vi "test_turbo2.vi"() -> ()   [LabVIEW 2018]
uses:
  <vilib>/addons/Modulation/Analog/support/mod_Set Error Source.vi
  <vilib>/addons/Modulation/Digital/Support/Common/Validators/mod_AWGN Validate.vi
  <vilib>/addons/Modulation/Digital/Impairments/subVIs/mod_createSeeds.vi
  <vilib>/addons/Modulation/Digital/Support/Common/Validators/mod_Validate Samples Per Symbol.vi
  <vilib>/addons/Modulation/Analog/support/Validators/mod_Validate Complex Waveform.vi
  <vilib>/addons/Modulation/Analog/support/Validators/mod_WFErrorHandler.vi
  <vilib>/addons/Modulation/Digital/Support/Common/Validators/mod_Generate Filter Coefficients Validate.vi
  <vilib>/addons/Modulation/Digital/General/subVIs/mod_Generate Filter Coefficients.vi
  <vilib>/addons/Modulation/Digital/General/MT Generate PSK System Parameters(M).vi
  <vilib>/addons/Modulation/Digital/General/subVIs/mod_Generate Bits PN Sequence.vi
  <vilib>/Analysis/1siggen.llb/Gaussian White Noise (obs 90).vi
  <vilib>/addons/Modulation/Digital/General/MT Apply Matched Filter (Generic).vi
  <vilib>/addons/Modulation/niDMT.lvlib
panel:
  out "message":i8[](array[numeric])
  out "#err":i32
  out "trial":i32
  in  "#trials":i32
  out "#bits":i32
  in  "Eb/N0":dbl=10.0 format="%.2f"
  out "BER":dbl
  out "Dec":i8[](array[numeric])
  out "sigma2":string
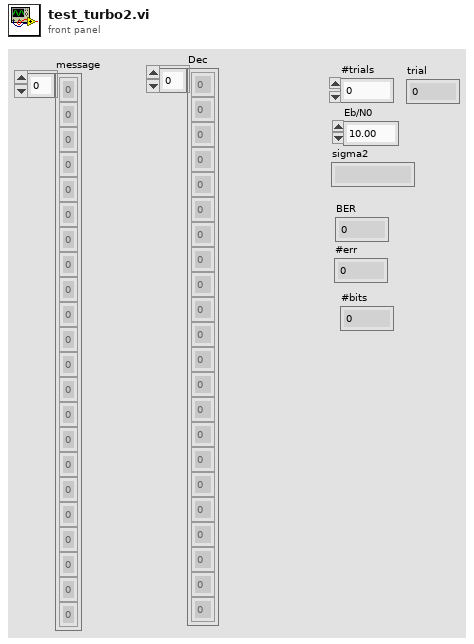
[diagram p1: front panel]
types:
  T1 = enum16{"none", "Raised Cosine", "Root Raised Cos", "Gaussian"}
  T2 = cluster{"samples per symbol (16)":i32, "symbol map":cdb[], "differential PSK":enum16{"disable", "enable"}, "PSK type":u16}
  T3 = typedef "niAMT.lvlib/Complex Data Waveform.ctl" = cluster{"t0":dbl, "dt":dbl, "Y":cdb[]}
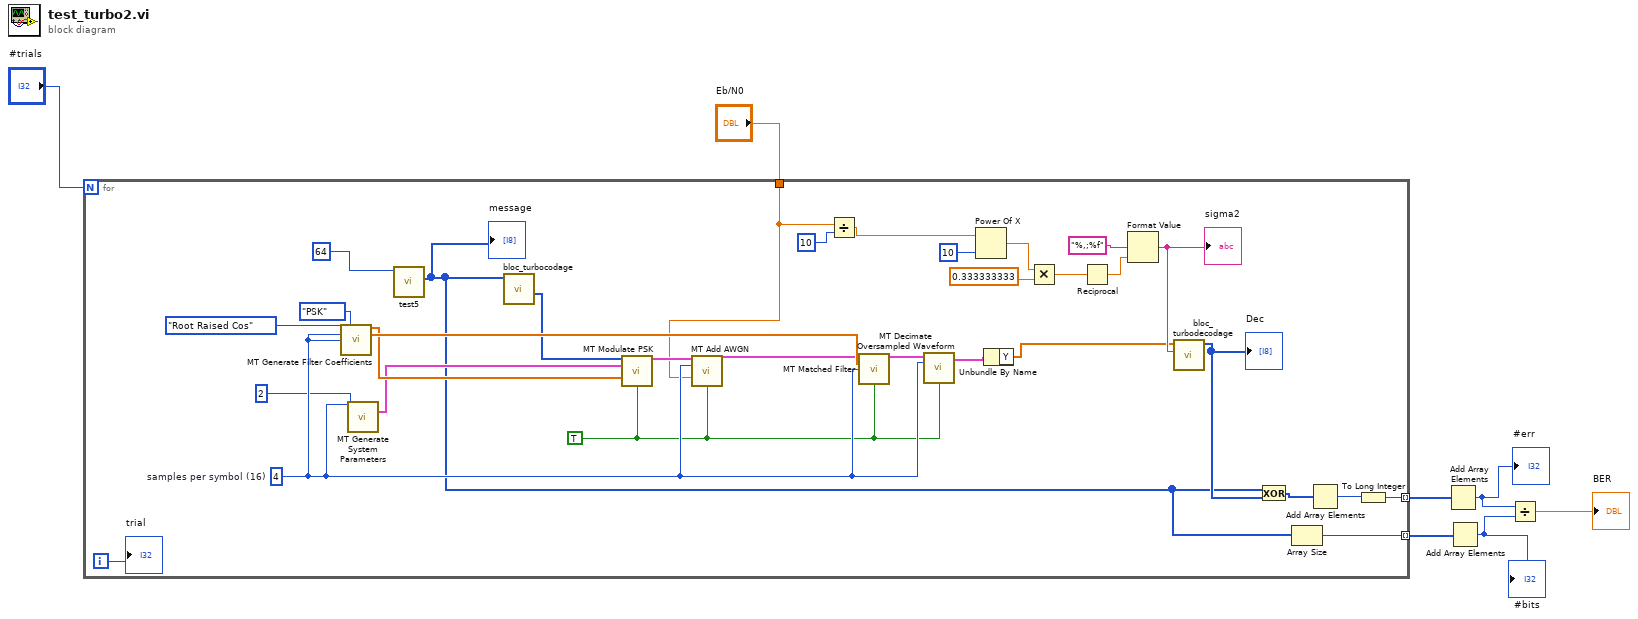
[diagram p0: block diagram]
diagram:
  n1 = for {
    N: "#trials" -> [_]
    tunnel: [w34] -> w6 mode=indexing
    tunnel: "Eb/N0" -> [w10]
    tunnel: [w25] -> w2 mode=indexing
    i -> [w27]
    w18 = 4  # samples per symbol (16)
    w14 = TRUE ("reset? (T)")
    n2 = call <vilib>:"MT Generate Filter Coefficients.vi"("pulse shaping filter (none)"=T1."Root Raised Cos", "modulation type"=enum16{"FSK", "PSK", "QAM", "MSK", "PAM", "ASK"}."PSK", "pulse shaping samples per symbol (16)"=w18, "matched samples per symbol (16)"=w18) -> ("pulse shaping filter coefficients"=w22:dbl[], "matched filter coefficients"=w24:dbl[])  [unwired: 9 in, 1 out]
    n3 = call-poly <vilib>:"MT Generate System Parameters.vi"("samples per symbol (16)"=w18, "M-PSK (4)"=2) -> ("PSK system parameters"=w19:T2)  [unwired: 11 in, 2 out]
    n4 = call "test5.vi"("k"=64) -> ("output bit stream"=w8:i8[])  [unwired: 9 in, 1 out]
    "message" <- w8
    n5 = call "bloc_turbocodage.vi"("Array in"=w8) -> ("output bit stream"=w21:i8[])  [unwired: 8 in, 2 out]
    n6 = call <vilib>:"MT Modulate PSK.vi"("input bit stream"=w21, "PSK system parameters"=w19, "pulse shaping filter coefficients"=w22, "reset? (T)"=w14) -> ("output complex waveform"=w23:T3)  [unwired: 9 in, 2 out]
    n7 = call <vilib>:"MT Add AWGN.vi"("input complex waveform"=w23, "samples per symbol (16)"=w18, "Eb/N0 (10 dB)"=w10, "reset? (T)"=w14) -> ("output complex waveform"=w11:T3)  [unwired: 9 in, 2 out]
    n8 = Divide(x=w10, y=10) -> (x/y=w29:dbl)
    n9 = call-poly <vilib>:"MT Matched Filter.vi"("input complex waveform"=w11, "matched filter coefficients"=w24, "samples per symbol (16)"=w18, "reset? (T)"=w14) -> ("output complex waveform"=w20:T3)  [unwired: 10 in, 1 out]
    n10 = call <vilib>:"MT Decimate Oversampled Waveform.vi"("input complex waveform"=w20, "decimation factor"=w18, "reset? (T)"=w14) -> ("output complex waveform"=w12:T3)  [unwired: 11 in, 1 out]
    n11 = Power Of X(1:10, 2:w29) -> (0:w30:dbl)
    n12 = Unbundle By Name(w12) -> ("Y"=w9:cdb[])
    n13 = Multiply(x=w30, y=0.333333333) -> (x*y=w38:dbl)
    n14 = Reciprocal(x=w38) -> (1/x=w36:dbl)
    n15 = Format Value(format string="%,;%f", value (0)=w36) -> (output string=w33:string)  [unwired: 1 in]
    "sigma2" <- w33
    n16 = call "bloc_turbodecodage.vi"("sigma2"=w33, "Array"=w9) -> ("output bit stream"=w32:i8[])  [unwired: 7 in, 2 out]
    "Dec" <- w32
    n17 = Exclusive Or(1:w32, 2:w8) -> (0:w35:i8[])
    n18 = Array Size(array=w8) -> (size(s)=w34:i32)
    n19 = Add Array Elements(numeric array=w35) -> (sum=w26:i8)
    n20 = To Long Integer(number=w26) -> (32bit integer=w25:i32)
    "trial" <- w27
  }
  n21 = Add Array Elements(numeric array=w2) -> (sum=w1:i32)
  "#err" <- w1
  n22 = Add Array Elements(numeric array=w6) -> (sum=w5:i32)
  "#bits" <- w5
  n23 = Divide(x=w1, y=w5) -> (x/y=→"BER":dbl)
